vi "Test_WriteItem_FloatKey_ReadWrongKeyValue_NotFound.vi"(8 "error in (no error)":errorcluster, 11 "TestCase in":refnum<class "TestComposedLookupTable.lvclass">) -> (0 "error out":errorcluster, 3 "TestCase out":refnum<class "TestComposedLookupTable.lvclass">)   [LabVIEW 2017, in "TestComposedLookupTable.lvclass"]
uses:
  TestComposedLookupTable.lvclass
  Source/LookupTable/LookupTable.lvclass/LookupTable.ctl
  de331345-f2dc-4322-a95c-a178be91e42b.vi
  d0b264f1-442b-48e7-b5c6-30e921ae893d.vi
  Source/LookupTable/Read Table Reference.vi
  de331345-f2dc-4322-a95c-a178be91e42b.vi/acc272e5-fd85-4fbb-b545-457fe05d68bd.vi
  d0b264f1-442b-48e7-b5c6-30e921ae893d.vi/cb16d91f-7dc1-4934-8d61-48f87877f0ed.vi
  Source/LookupTable/LookupTable.lvclass
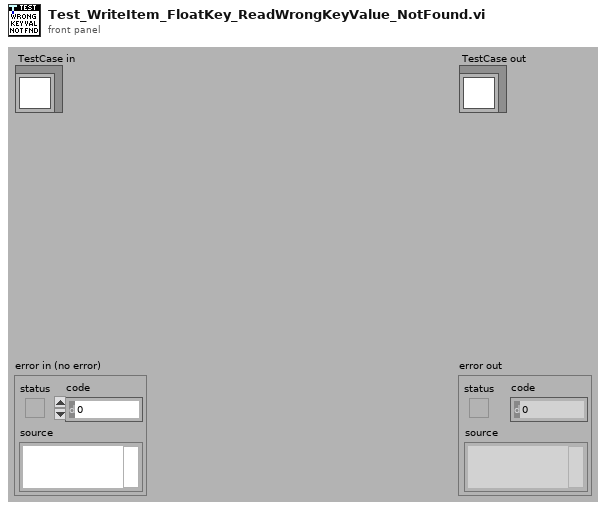
[diagram p1: front panel]
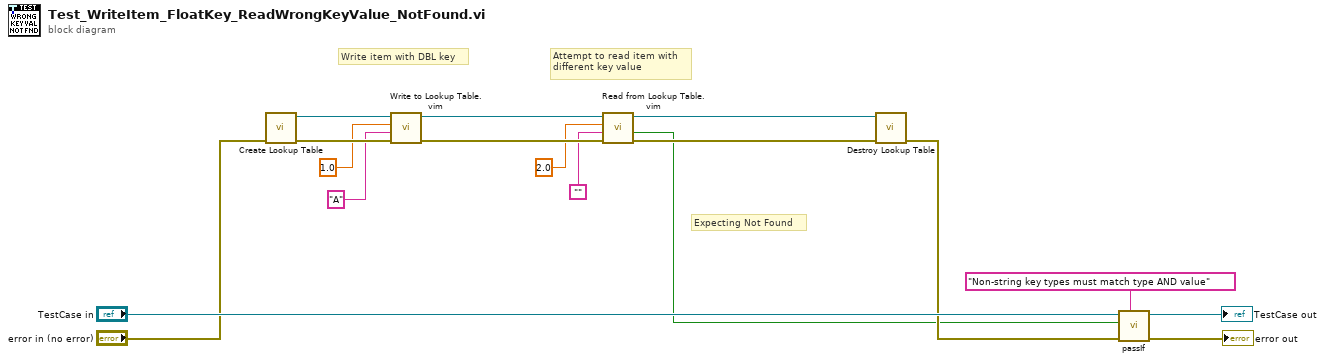
[diagram p0: block diagram]
diagram:
  # "Expecting Not Found"
  # "Attempt to read item with\ndifferent key value"
  # "Write item with DBL key"
  n1 = call "Create Lookup Table.vi"("error in (no error)"="error in (no error)") -> ("error out"=w17:errorcluster, "LookupTable Reference"=w9:refnum<data-value>)  [unwired: 9 in]
  n2 = call "Write to Lookup Table.vim"("error in (no error)"=w17, "Item"="A" ("Item Name"), "Item Name"=1.0, "LookupTable Reference"=w9) -> ("error out"=w11:errorcluster, "LookupTable Reference Out"=w7:refnum<data-value>)  [unwired: 5 in, 1 out]
  n3 = call "Read from Lookup Table.vim"("error in (no error)"=w11, "Type"="", "Item Name"=2.0, "LookupTable Reference"=w7) -> ("error out"=w8:errorcluster, "Not Found?"=w1:bool, "LookupTable Reference Out"=w12:refnum<data-value>)  [unwired: 4 in, 1 out]
  n4 = call "Destroy Lookup Table.vi"("error in (no error)"=w8, "LookupTable Reference"=w12) -> ("error out"=w10:errorcluster)  [unwired: 9 in]
  n5 = call-dynamic "passIf.vi"("custom report message (\"\")"="Non-string key types must match type AND value" ("message (\"\")"), "error in (no error)"=w10, "pass"=w1, "TestCase in"="TestCase in") -> ("error out"=→"error out":errorcluster, "TestCase out"=→"TestCase out":refnum<class "TestComposedLookupTable.lvclass">)  [unwired: 6 in]
